vi "move.vi"   [LabVIEW 2010]
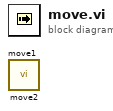
[diagram p0: block diagram]
diagram:
  n1 = call "move2.vi"() -> ()  [unwired: 7 in, 1 out]
  n2 = call "move1.vi"() -> ()  [unwired: 7 in, 1 out]
